vi "run.vi"(11 "wait action in":refnum<class "wait action.lvclass">) -> (2 "result":refnum<class "result.lvclass">, 3 "wait action out":refnum<class "wait action.lvclass">)   [LabVIEW 2013, in "wait action.lvclass"]
uses:
  wait action.lvclass
  result/result.lvclass
  wait action.lvclass/wait action.ctl
  task/task.lvclass/task.ctl
  task token/null task token.lvclass
  task/task.lvclass
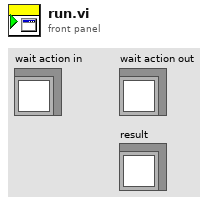
[diagram p1: front panel]
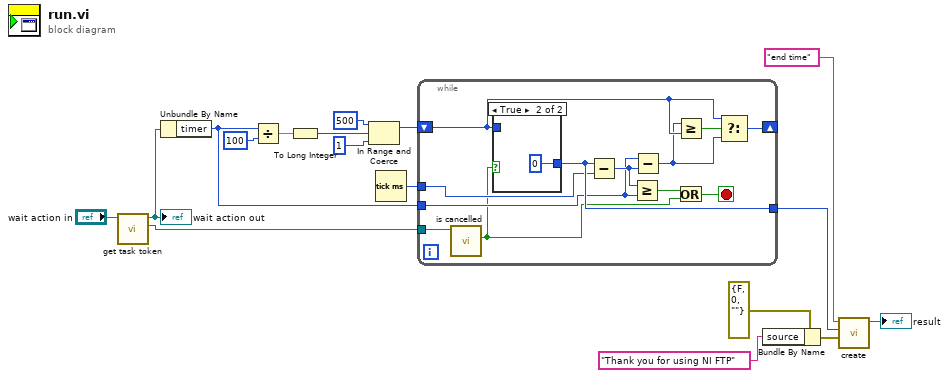
[diagram p0: block diagram]
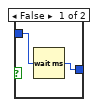
[diagram p2: hidden frame]
diagram:
  n1 = call "get task token.vi"("task in"="wait action in") -> ("task token"=w1:refnum<class "null task token.lvclass">, "task out"=w2:refnum<class "wait action.lvclass">)  [unwired: 9 in]
  "wait action out" <- w2
  n2 = Unbundle By Name(w2) -> ("timer"=w4:i32)
  n3 = Divide(x=w4, y=u32 100) -> (x/y=w11:dbl)
  n4 = To Long Integer(number=w11) -> (32bit integer=w10:i32)
  n5 = In Range and Coerce(upper limit=500, x=w10, lower limit=1) -> (coerced(x)=w7:i32)  [unwired: 1 out]
  n6 = Tick Count (ms)() -> (millisecond timer value=w13:u32)
  n7 = while {
    tunnel: [w28] -> w15
    tunnel: w1 -> [w29]
    tunnel: w13 -> [w27]
    tunnel: w4 -> [w23]
    shift-right: [w20] -> _
    shift-left: w7 -> [w21]
    stop <- w26 stop-if-true
    n8 = call-dynamic "is cancelled.vi"("null task token in"=w29) -> ("cancelled?"=w18:bool)  [unwired: 9 in, 1 out]
    n9 = case shown="True" w18 {
      tunnel: [w31 u32 0 ("millisecond timer value")] -> w28
      tunnel: w21 -> [w30 _]
      frame False {
        n10 = Wait (ms)(milliseconds to wait=w30) -> (millisecond timer value=w31:u32)
      }
      frame True {
      }
    }
    n11 = Subtract(x=w28, y=w27) -> (x-y=w24:u32)
    n12 = Greater Or Equal?(x=w24, y=w23) -> (x >= y?=w25:bool)
    n13 = Subtract(x=w23, y=w24) -> (x-y=w19:u32)
    n14 = Greater Or Equal?(x=w19, y=w21) -> (x >= y?=w22:bool)
    n15 = Or(x=w25, y=w18) -> (x .or. y?=w26:bool)
    n16 = Select(t=w21, s=w22, f=w19) -> (s? t:f=w20:u32)
  }
  n17 = Bundle By Name(cluster=errorcluster {"status"=FALSE, "code"=0, "source"=""} ("error in (no error)"), "source"="Thank you for using NI FTP") -> (w16:errorcluster)
  n18 = call "create.vi"("error"=w16, "data"=w15, "data ID"="end time") -> ("result out"=→"result":refnum<class "result.lvclass">)  [unwired: 8 in]
